vi "K avg filter (no using FIR vi).vi"(9 "num avg":i32=10, 11 "input":dbl) -> (3 "output":dbl)   [LabVIEW 2018]
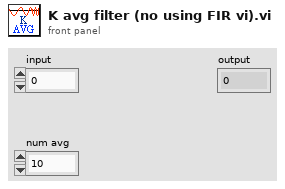
[diagram p1: front panel]
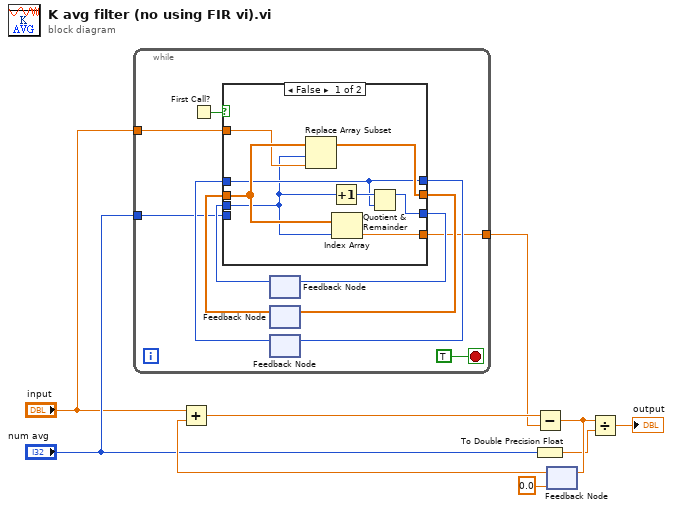
[diagram p0: block diagram]
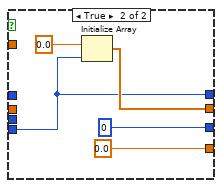
[diagram p2: hidden frame]
diagram:
  n1 = while {
    tunnel: "num avg" -> [w13]
    tunnel: "input" -> [w11]
    tunnel: [w10] -> w3
    stop <- TRUE stop-if-true
    n2 = First Call?() -> (First Call?: T/F=w20:bool)
    n3 = feedback #1() -> (w18:i32)  [unwired: 1 in]
    n4 = feedback #2() -> (w16:dbl[])  [unwired: 1 in]
    n5 = feedback #3() -> (w14:i32)  [unwired: 1 in]
    n6 = case shown="False" w20 {
      tunnel: [w27 w33] -> w17
      tunnel: w16 -> [w28 _]
      tunnel: [w24 0 ("index")] -> w19
      tunnel: w18 -> [w22 _]
      tunnel: [w25 w29] -> w15
      tunnel: w14 -> [w25 _]
      tunnel: w11 -> [w23 _]
      tunnel: [w21 0.0 ("input")] -> w10
      tunnel: w13 -> [_ w29]
      frame False {
        n7 = Replace Array Subset(array=w28, new element=w23, index=w22) -> (w27:dbl[])
        n8 = Increment(x=w22) -> (x+1=w26:i32)
        n9 = Index Array(array=w28, index=w22) -> (element=w21:dbl)
        n10 = Quotient & Remainder(x=w26, y=w25) -> (x-y*floor(x/y)=w24:i32)  [unwired: 1 out]
      }
      frame True {
        n11 = Initialize Array(0.0 ("input"), w29) -> (w33:dbl[])
      }
    }
    n12 = feedback-in #1(w19) -> ()
    n13 = feedback-in #2(w17) -> ()
    n14 = feedback-in #3(w15) -> ()
  }
  n15 = To Double Precision Float(number="num avg") -> (double precision float=w5:dbl)
  n16 = feedback #4(0.0) -> (w8:dbl)
  n17 = Add(x="input", y=w8) -> (x+y=w9:dbl)
  n18 = Subtract(x=w9, y=w3) -> (x-y=w6:dbl)
  n19 = feedback-in #4(w6) -> ()
  n20 = Divide(x=w6, y=w5) -> (x/y=→"output":dbl)
